vi "Constructor.vi"(8 "error in":errorcluster, 9 "Value":T1, 10 "Name":string, 11 "Measure in":refnum<class "MeasureKind.lvclass">) -> (0 "error out":errorcluster, 3 "Measure out":refnum<class "MeasureKind.lvclass">)   [LabVIEW 2021, in "ProligentXMLGenerator.lvlib" / "MeasureKind.lvclass"]
uses:
  MeasureKind.lvclass
  MeasureKind.lvclass/MeasureKind.ctl
  Attribute/Attribute.lvclass
  C:/Projects/proligent-xml-generator-labview/src/ProligentXMLGenerator/Base/Attribute/Attribute.lvclass
  C:/Projects/proligent-xml-generator-labview/src/ProligentXMLGenerator/Base/MeasureKind/MeasureKind.lvclass
  Value.ctl
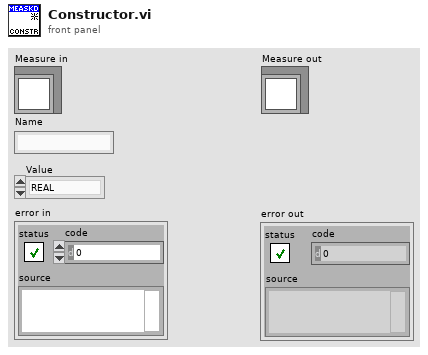
[diagram p1: front panel]
types:
  T1 = typedef "ProligentXMLGenerator.lvlib/MeasureKind.lvclass/Value.ctl" = enum16{"REAL", "BOOL", "INTEGER", "STRING", "DATETIME"}
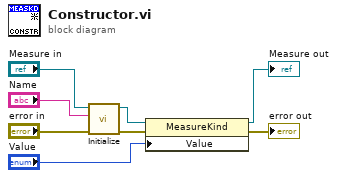
[diagram p0: block diagram]
diagram:
  n1 = call "Initialize.vi"("error in"="error in", "Name"="Name", "Attribute in"="Measure in") -> ("error out"=w4:errorcluster, "Attribute out"=w3:refnum<class "MeasureKind.lvclass">)  [unwired: 7 in]
  n2 = property on="Property Node" class="MeasureKind"(reference=w3, error in=w4, "Value"="Value") -> (reference out=→"Measure out":refnum<class "MeasureKind.lvclass">, error out=→"error out":errorcluster)
